vi "Wait_Server_Answer (SubVI).vi"(11 "TCP Network Connection in":refnum<k5>) -> (0 "total_message":string, 2 "data out":string, 3 "TCP Network Connection out":refnum<k5>, 4 "Tag":string)   [LabVIEW 2015]
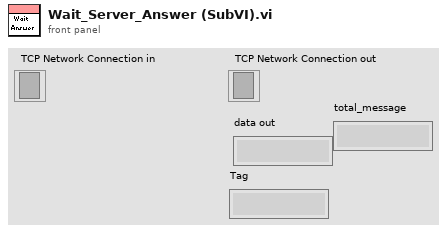
[diagram p1: front panel]
types:
  T1 = enum16{"Standard", "Buffered", "CRLF", "Immediate"}
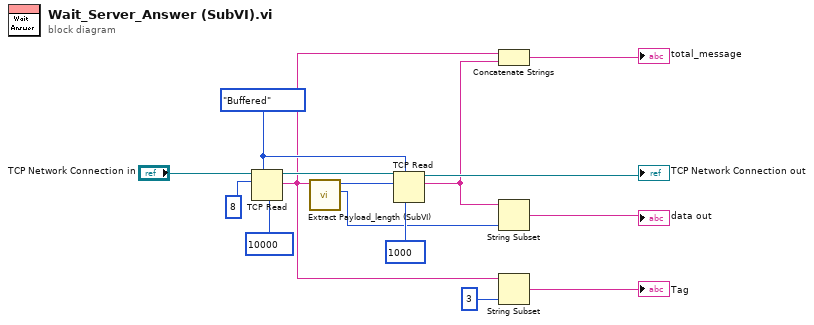
[diagram p0: block diagram]
diagram:
  w13 = T1."Buffered" ("mode (standard)")
  n1 = TCP Read(connection ID="TCP Network Connection in", bytes to read=8, 7:w13, 9:10000 ("timeout ms (25000)")) -> (connection ID out=w11:refnum<k5>, data out=w1:string)  [unwired: 1 in, 1 out]
  n2 = call "Extract Payload_length (SubVI).vi"("data in"=w1) -> ("Payload_length"=w7:u32, "Total_Length"=w14:i32)  [unwired: 8 in, 1 out]
  n3 = TCP Read(connection ID=w11, bytes to read=w14, 7:w13, 9:1000 ("timeout ms (25000)")) -> (connection ID out=→"TCP Network Connection out":refnum<k5>, data out=w4:string)  [unwired: 1 in, 1 out]
  n4 = Concatenate Strings(w1, w4) -> (→"total_message":string)
  n5 = String Subset(string=w4, length (rest)=w7) -> (substring=→"data out":string)  [unwired: 1 in]
  n6 = String Subset(string=w1, length (rest)=3 ("length (rest)")) -> (substring=→"Tag":string)  [unwired: 1 in]
